vi "Add File.vi"(8 "error in (no error)":errorcluster, 9 "Insert in front":bool=TRUE, 10 "File Path":path, 11 "Plot in":refnum<class "Plot.lvclass">) -> (0 "error out":errorcluster, 2 "Success":bool, 3 "Plot out":refnum<class "Plot.lvclass">)   [LabVIEW 2015, in "Plot.lvclass"]
uses:
  Plot.lvclass
  <vilib>/ActorFramework/Actor/Actor.lvclass/Actor.ctl
  <vilib>/ActorFramework/Message Enqueuer/Message Enqueuer.lvclass/Message Enqueuer.ctl
  Plot Messages/Add file Msg/Add file Msg.lvclass/Add file Msg.ctl
  <vilib>/ActorFramework/Message Enqueuer/Init from Existing Queue.vi
  <vilib>/ActorFramework/Time-Delayed Send Message/Time-Delayed Send Message.vi
  <vilib>/ActorFramework/Message Enqueuer/Message Enqueuer.lvclass
  Plot Messages/Add file Msg/Add file Msg.lvclass
  <vilib>/ActorFramework/Actor/Actor.lvclass
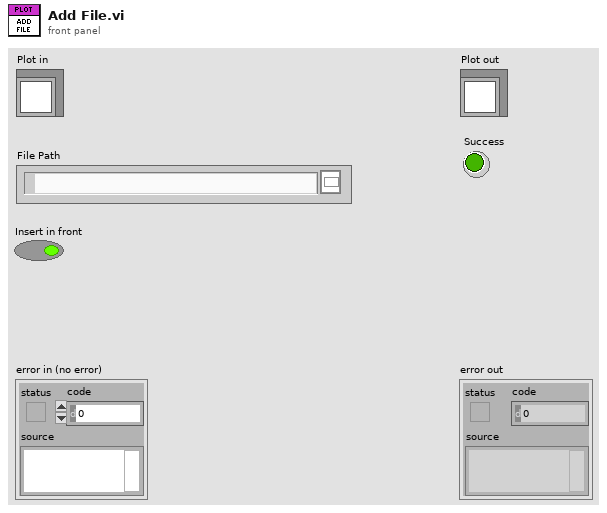
[diagram p1: front panel]
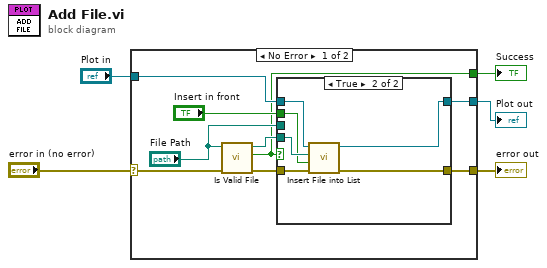
[diagram p0: block diagram]
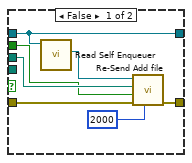
[diagram p2: hidden frame]
diagram:
  n1 = case shown="No Error" "error in (no error)" {
    selector: "error in (no error)" -> [w11 w29]
    tunnel: [w12 w29] -> w2
    tunnel: [w13 w28] -> w3
    tunnel: "Plot in" -> [w14 w28]
    tunnel: [w6 _] -> w1
    frame No Error {
      n2 = call "Is Valid File.vi"("Error In"=w11, "File"="File Path") -> ("Error Out"=w10:errorcluster, "Valid file"=w6:bool, "File out"=w9:path)  [unwired: 7 in]
      n3 = case shown="True" w6 {
        tunnel: w10 -> [w20 w24]
        tunnel: w14 -> [w18 w25]
        tunnel: [w18 w23] -> w13
        tunnel: [w19 w22] -> w12
        tunnel: w9 -> [_ w27]
        tunnel: "File Path" -> [w17 _]
        tunnel: "Insert in front" -> [w16 w26]
        frame False {
          n4 = call <vilib>:"Read Self Enqueuer.vi"("Actor"=w18) -> ("Self Enqueuer"=w21:refnum<class "Message Enqueuer.lvclass">)  [unwired: 10 in]
          n5 = call "Re-Send Add file.vi"("Milliseconds To Wait"=2000, "error in (no error)"=w20, "Insert in front"=w16, "File Path Control"=w17, "Message Enqueuer"=w21) -> ("error out"=w19:errorcluster)  [unwired: 5 in, 1 out]
        }
        frame True {
          n6 = call-dynamic "Insert File into List.vi"("error in (no error)"=w24, "Insert in front"=w26, "File"=w27, "Plot in"=w25) -> ("error out"=w22:errorcluster, "Plot out"=w23:refnum<class "Plot.lvclass">)  [unwired: 6 in]
        }
      }
    }
    frame Error {
    }
  }
  "error out" <- w2
  "Plot out" <- w3
  "Success" <- w1
